vi "QP_Solver-minerror.vi"(4 "DesiredFM":dbl[](array[numeric]), 6 "Constants HL":T1={"Frame Points"=[], "Brace Points in P"=[], "QP_lb"=[], "QP_ub"=[], "Q for QP"=[], "nMotors"=0, "QP stopping criteria"={"function tolerance"=1e-08, "parameter tolerance"=1000000.0, "max iterations"=10000, "max function calls"=10000, "gradient tolerance"=1000000.0, "max time (sec)"=-1.0}, "MotorsPos_wrt_Markers"=[], "nMotors 1"=0, "nMotors 2"=0, "MotorsPos_wrt_Markers pel"=[], "Frame Points_pel"=[], "Brace Points in P_pel"=[], "QP_lb pel"=[], "QP_ub pel"=[], "Q for QP pel"=[], "MotorsPos_wrt_Markers knees"=[], "nMotors 3"=0}, 7 "A matrix":T3) -> (1 "error out":errorcluster, 2 "minT":dbl[](array[numeric]))   [LabVIEW 2017]
uses:
  <vilib>/Analysis/Matrix/Datatypes/RealMatrix.ctl
  typeDef/constants_HL.ctl
  <vilib>/gmath/NumericalOptimization/stopping criteria.ctl
  <vilib>/Analysis/7linalg.llb/Create Special Real Matrix.vi
  <vilib>/Analysis/Matrix/Numeric/Conversions/Array To Matrix - RA.vi
  <vilib>/Analysis/Matrix/Numeric/Multiply/Multiply - RM,RM.vi
  <vilib>/Analysis/Matrix/Numeric/Multiply/Multiply - R,RM.vi
  <vilib>/Analysis/Matrix/Numeric/Add/Add - RM,RM.vi
  <vilib>/gmath/NumericalOptimization/Quadratic Programming IP.vi
  <vilib>/gmath/NI_Gmath.lvlib
  <vilib>/Analysis/NI_AALPro.lvlib
  <vilib>/Analysis/Matrix/NI_Matrix.lvlib
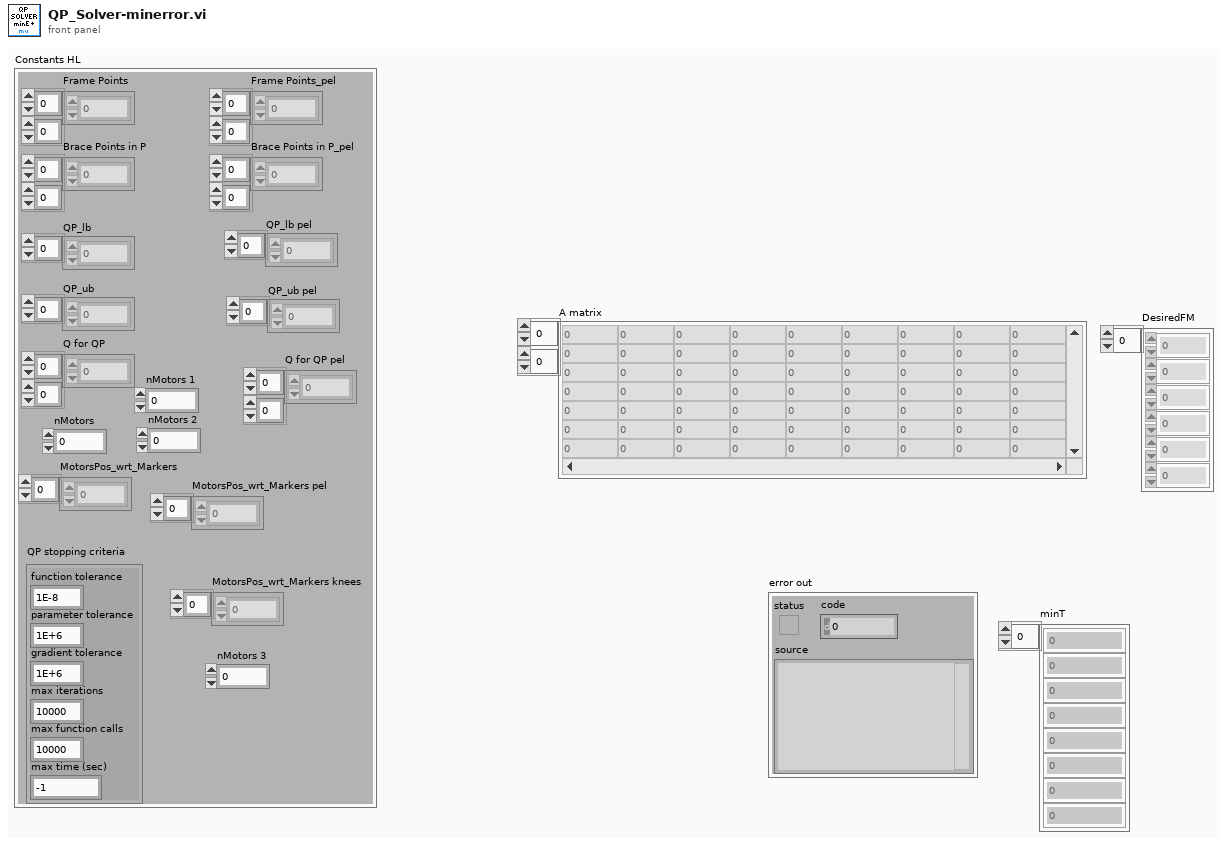
[diagram p1: front panel]
types:
  T1 = typedef "constants_HL.ctl" = cluster{"Frame Points":dbl[][], "Brace Points in P":dbl[][], "QP_lb":dbl[], "QP_ub":dbl[], "Q for QP":dbl[][], "nMotors":i32, "QP stopping criteria":T2, "MotorsPos_wrt_Markers":i32[], "nMotors 1":i32, "nMotors 2":i32, "MotorsPos_wrt_Markers pel":i32[], "Frame Points_pel":dbl[][], "Brace Points in P_pel":dbl[][], "QP_lb pel":dbl[], "QP_ub pel":dbl[], "Q for QP pel":dbl[][], "MotorsPos_wrt_Markers knees":i32[], "nMotors 3":i32}
  T2 = typedef "NI_Gmath.lvlib/stopping criteria.ctl" = cluster{"function tolerance":dbl, "parameter tolerance":dbl, "max iterations":i32, "max function calls":i32, "gradient tolerance":dbl, "max time (sec)":dbl}
  T3 = typedef "NI_Matrix.lvlib/RealMatrix.ctl" = dbl[][]
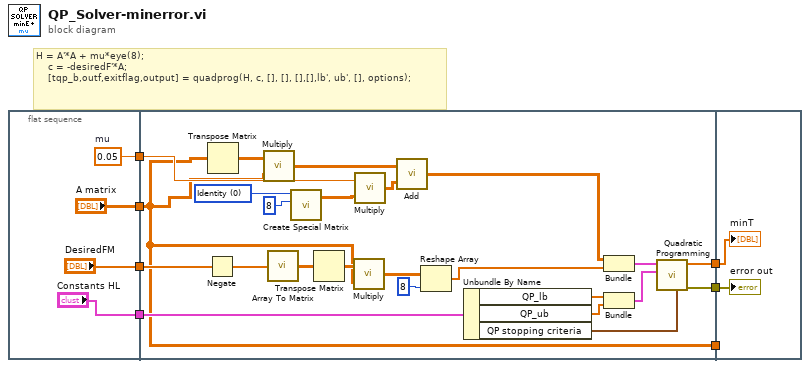
[diagram p0: block diagram]
diagram:
  # "H = A'*A + mu*eye(8);\n    c = -desiredF'*A;\n    [tqp_b,outf,exitflag,output] = quadprog(H, c, [], [], [],[],lb', ub', [], options);"
  n1 = flat-sequence {
    tunnel: ["Constants HL"] -> w7
    tunnel: [w11] -> w6
    tunnel: ["A matrix"] -> w5
    tunnel: ["DesiredFM"] -> w4
    tunnel: w7 -> [w35]
    tunnel: w6 -> [w29]
    tunnel: w5 -> [w12]
    tunnel: w4 -> [w23]
    tunnel: [w14] -> w3
    tunnel: [w13] -> w2
    tunnel: [w12] -> w1
    tunnel: w3 -> [w36]
    tunnel: w2 -> [w37]
    tunnel: w1 -> [_]
    frame #0 {
      w11 = 0.05  # mu
    }
    frame #1 {
      w31 = 0 items=["Identity", "Diagonal", "Toeplitz", "Vandermonde", "Companion", "Hankel", "Hadamard", "Wilkinson", "Hilbert", "Inverse Hilbert", "Rosser", "Pascal"] ("matrix type")
      n2 = Negate(x=w23) -> (-x=w22:dbl[])
      n3 = Transpose Matrix(1:w12) -> (0:w26:T3)
      n4 = call-poly <vilib>:"Multiply.vi"("Real Matrix B"=w12, "Real Matrix A"=w26) -> ("A * B"=w25:T3)
      n5 = call-poly <vilib>:"Array To Matrix.vi"("Real 1D Array"=w22) -> ("Real Matrix (Column Vector)"=w21:T3)
      n6 = call-poly <vilib>:"Create Special Matrix.vi"("matrix type"=w31, "matrix size"=8) -> ("Special Matrix"=w28:T3)  [unwired: 3 in, 1 out]
      n7 = Transpose Matrix(1:w21) -> (0:w20:T3)
      n8 = call-poly <vilib>:"Multiply.vi"("Real Matrix B"=w12, "Real Matrix A"=w20) -> ("A * B"=w18:T3)
      n9 = call-poly <vilib>:"Multiply.vi"("Real Matrix A"=w28, "Real Scalar c"=w29) -> ("c * A"=w27:T3)
      n10 = call-poly <vilib>:"Add.vi"("Real Matrix B"=w27, "Real Matrix A"=w25) -> ("A + B"=w24:T3)
      n11 = Reshape Array(w18, 8 ("dimension size")) -> (w16:dbl[])
      n12 = Unbundle By Name(w35) -> ("QP_lb"=w34:dbl[], "QP_ub"=w33:dbl[], "QP stopping criteria"=w15:T2)
      n13 = Bundle("A + B"=w24, "A * B"=w16) -> (w19:cluster{"A + B":T3, "A * B":dbl[]})  [unwired: 1 in]
      n14 = Bundle("QP_lb"=w34, "QP_ub"=w33) -> (w32:cluster{"QP_lb":dbl[], "QP_ub":dbl[]})  [unwired: 1 in]
      n15 = call-poly <vilib>:"Quadratic Programming.vi"("stopping criteria"=w15, "parameter bounds"=w32, "objective function"=w19) -> ("error out"=w13:errorcluster, "minimum"=w14:dbl[])  [unwired: 5 in, 2 out]
    }
    frame #2 {
      "minT" <- w36
      "error out" <- w37
    }
  }
